vi "Scan Insert Type_RegExp.vi"(10 "Pattern In":string) -> (1 "OK?":bool, 3 "Insert Type Out":string)   [LabVIEW 2026]
panel:
  out "First Scan?":bool
  in  "Case Constant\n(See Context Help)":bool
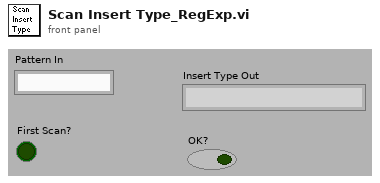
[diagram p1: front panel]
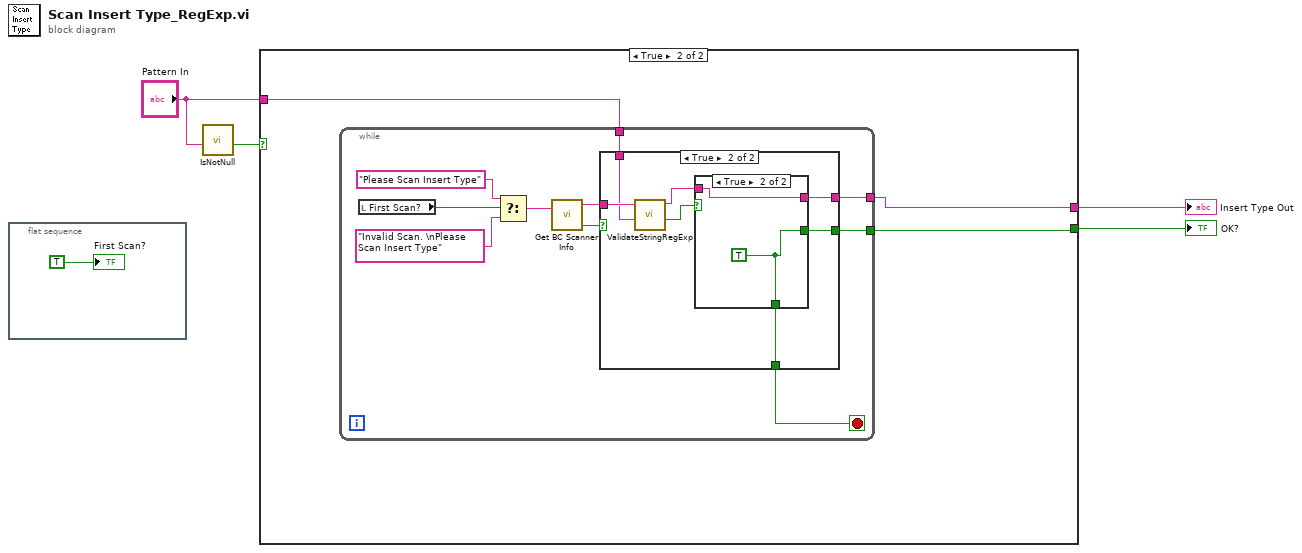
[diagram p0: block diagram]
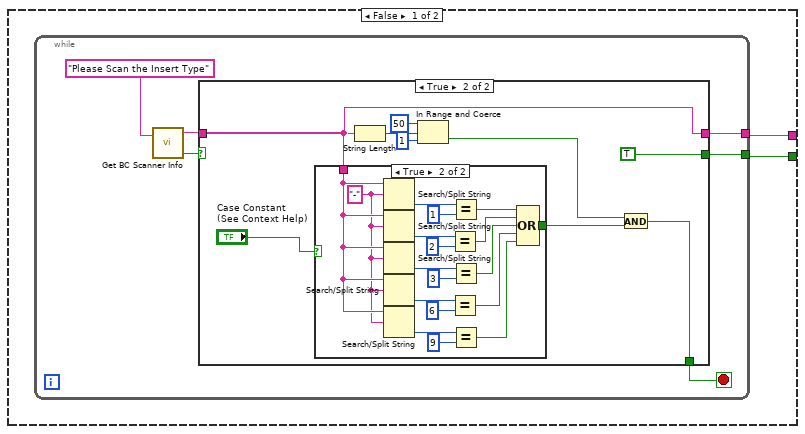
[diagram p2: hidden frame]
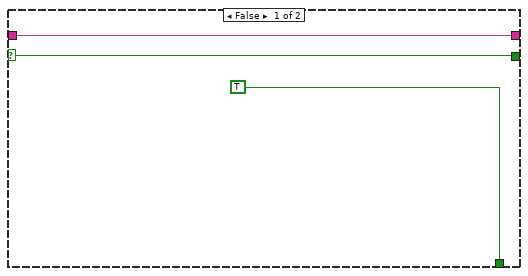
[diagram p3: hidden frame]
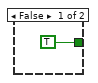
[diagram p4: hidden frame]
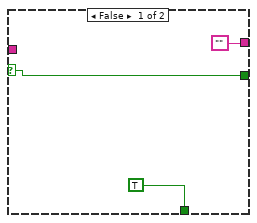
[diagram p5: hidden frame]
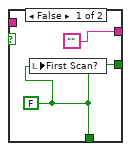
[diagram p6: hidden frame]
diagram:
  n1 = flat-sequence {
    frame #0 {
      "First Scan?" <- TRUE
    }
  }
  n2 = call "IsNotNull.vi"("String In"="Pattern In") -> ("Boolean Out"=w2:bool)  [unwired: 10 in]
  n3 = case shown="True" w2 {
    tunnel: [w7 w47] -> w4
    tunnel: [w6 w46] -> w3
    tunnel: "Pattern In" -> [_ w45]
    frame False {
      n4 = while {
        tunnel: [w8] -> w6
        tunnel: [w10] -> w7
        stop <- w9 stop-if-true
        n5 = call "Get BC Scanner Info.vi"("Prompt"="Please Scan the Insert Type") -> ("Info Out"=w11:string, "OK"=w12:bool)  [unwired: 2 in]
        n6 = case shown="True" w12 {
          selector: w12 -> [w14 _]
          tunnel: w11 -> [w16 w21]
          tunnel: [w16 w21] -> w10
          tunnel: [TRUE ("OK") w20] -> w9
          tunnel: [w14 TRUE ("OK")] -> w8
          frame False {
          }
          frame True {
            n7 = case shown="True" "Case Constant\n(See Context Help)" {
              tunnel: w21 -> [_ w34]
              tunnel: [TRUE w27] -> w19
              frame False {
              }
              frame True {
                w33 = "-" ("search string/char (-)")
                n8 = Search/Split String(string=w34, search string/char (-)=w33) -> (offset of match=w44:i32)  [unwired: 1 in, 2 out]
                n9 = Search/Split String(string=w34, search string/char (-)=w33) -> (offset of match=w43:i32)  [unwired: 1 in, 2 out]
                n10 = Search/Split String(string=w34, search string/char (-)=w33) -> (offset of match=w37:i32)  [unwired: 1 in, 2 out]
                n11 = Search/Split String(string=w34, search string/char (-)=w33) -> (offset of match=w38:i32)  [unwired: 1 in, 2 out]
                n12 = Search/Split String(string=w34, search string/char (-)=w33) -> (offset of match=w36:i32)  [unwired: 1 in, 2 out]
                n13 = Equal?(x=w43, y=2) -> (x = y?=w31:bool)
                n14 = Equal?(x=w38, y=6) -> (x = y?=w29:bool)
                n15 = Equal?(x=w44, y=1) -> (x = y?=w32:bool)
                n16 = Equal?(x=w37, y=3) -> (x = y?=w30:bool)
                n17 = Equal?(x=w36, y=9) -> (x = y?=w28:bool)
                n18 = Compound Arithmetic op=OR(w32, w31, w30, w29, w28) -> (w27:bool)
              }
            }
            n19 = String Length(string=w21) -> (length=w24:i32)
            n20 = In Range and Coerce(upper limit=50, x=w24, lower limit=1) -> (In Range?=w18:bool)  [unwired: 1 out]
            n21 = And(x=w18, y=w19) -> (x .and. y?=w20:bool)
          }
        }
      }
    }
    frame True {
      n22 = while {
        tunnel: [w51] -> w47
        tunnel: [w50] -> w46
        tunnel: w45 -> [w48]
        stop <- w49 stop-if-true
        n23 = local read "First Scan?"() -> (w55:bool)
        n24 = Select(t="Please Scan Insert Type", s=w55, f="Invalid Scan. \nPlease Scan Insert Type") -> (s? t:f=w54:string)
        n25 = call "Get BC Scanner Info.vi"("Prompt"=w54) -> ("Info Out"=w52:string, "OK"=w53:bool)  [unwired: 2 in]
        n26 = case shown="True" w53 {
          selector: w53 -> [w59 _]
          tunnel: w52 -> [_ w64]
          tunnel: ["" w67] -> w51
          tunnel: [w59 w66] -> w50
          tunnel: [TRUE w65] -> w49
          tunnel: w48 -> [_ w63]
          frame False {
          }
          frame True {
            n27 = call "ValidateStringRegExp.vi"("Pattern In"=w63, "String To Match"=w64) -> ("Match Found"=w61:bool, "String Out"=w62:string)  [unwired: 8 in]
            n28 = case shown="True" w61 {
              tunnel: ["" w70] -> w67
              tunnel: [w69 w71] -> w66
              tunnel: [w69 w71] -> w65
              tunnel: w62 -> [_ w70]
              frame False {
                w69 = FALSE
                n29 = local write "First Scan?"(w69) -> ()
              }
              frame True {
                w71 = TRUE
              }
            }
          }
        }
      }
    }
  }
  "Insert Type Out" <- w4
  "OK?" <- w3
